vi "Transfer From Target Status.vi"(8 "error in":errorcluster, 10 "Reply Payload":T1) -> (0 "error out":errorcluster)   [LabVIEW 2015, in "LV-WinSCP.lvlib"]
doc: "This request allows transferring a file or an entire folder from the target to the local PC.\nFile transfer status might take longer than the module timeout. A brodacast is then also fired with the transfer status when it finishes. Therefore, asking for a reply is optional.\nA connection to the target must be done before using this request.\n_____\nCreated using DQMH Event Scripter 6.1.0.128."
uses:
  LV-WinSCP.lvlib
  Get Items From Target (Reply Payload)--cluster.ctl
  Classes/FileTransfer/FileAndDestination.ctl
  Classes/FileTransfer/TransferExceptionDescription.ctl
  Classes/FileTransfer/FileTransfer.lvclass
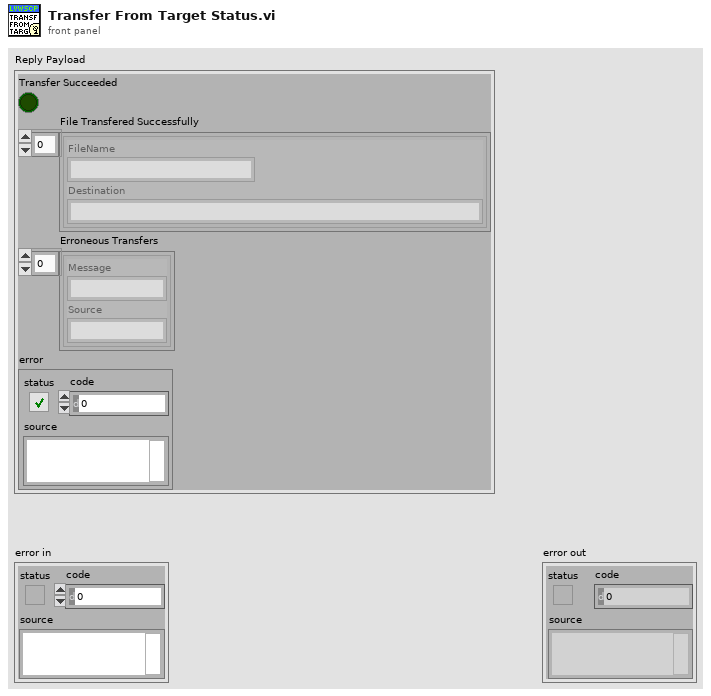
[diagram p1: front panel]
types:
  T1 = typedef "LV-WinSCP.lvlib/Get Items From Target (Reply Payload)--cluster.ctl" = cluster{"Transfer Succeeded":bool, "File Transfered Successfully":T2[], "Erroneous Transfers":T3[], "error":errorcluster}
  T2 = typedef "WinSCP.lvlib/FileTransfer.lvclass/FileAndDestination.ctl" = cluster{"FileName":string, "Destination":string}
  T3 = typedef "WinSCP.lvlib/FileTransfer.lvclass/TransferExceptionDescription.ctl" = cluster{"Message":string, "Source":string}
  T4 = typedef "LV-WinSCP.lvlib/Broadcast Events--cluster.ctl" = cluster{"Module Did Init":refnum<user-event>, "Status Updated":refnum<user-event>, "Error Reported":refnum<user-event>, "Module Did Stop":refnum<user-event>, "Update Module Execution Status":refnum<user-event>, "Transfer From Target Status":refnum<user-event>}
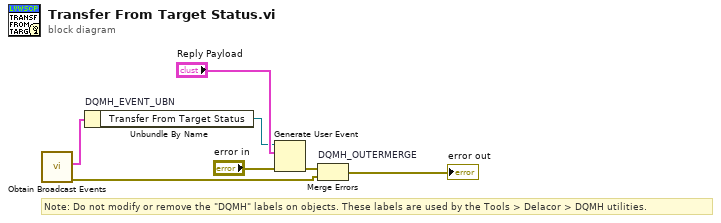
[diagram p0: block diagram]
diagram:
  # "Note: Do not modify or remove the \"DQMH\" labels on objects. These labels are used by the Tools > Delacor > DQMH utilities."
  n1 = call "Obtain Broadcast Events.vi"() -> ("error out"=w2:errorcluster, "LV-WinSCP Broadcast Events"=w1:T4)  [unwired: 10 in]
  n2 = Unbundle By Name "DQMH_EVENT_UBN"(w1) -> ("Transfer From Target Status"=w4:refnum<user-event>)
  n3 = Generate User Event(user event=w4, event data cluster="Reply Payload", error in="error in") -> (error out=w3:errorcluster)  [unwired: 1 in, 1 out]
  n4 = Merge Errors "DQMH_OUTERMERGE"(w3, w2) -> (→"error out":errorcluster)
